vi "Teleop.vi"(10 "Match Info":T1={"Autonomous Elapsed Seconds"=0.0, "TeleOp Elapsed Seconds"=0.0, "Disabled Elapsed Seconds"=0.0, "Visited Autonomous"=FALSE, "Visited TeleOp"=FALSE, "Visited Disabled"=FALSE, "Autonomous Settings"={"Autonomous Style"=enum."Independent", "VI Refnum"=refnum}}, 11 "Call Context":T2) -> ()   [LabVIEW 2016]
doc: "This VI is called for each TeleOp packet received from the DS where the robot is not disabled. It is often used to read from the joysticks and update I/O or to update setpoints for timed control loops. It should complete and return within 20 milliseconds or it may miss DS packets."
uses:
  <vilib>/Rock Robotics/WPI/DriverStation/WPI_DriverStationDerivedRobotMode.ctl
  <vilib>/Rock Robotics/WPI/DriverStation/WPI_DriverStationMatch Info.ctl
  <vilib>/Rock Robotics/WPI/Utilities/WPI_GetSetVariantRefNum.vi
  <vilib>/Rock Robotics/Network Tables/NT Write Boolean Array.vi
  <vilib>/Rock Robotics/Network Tables/NT Write Numeric Array.vi
  <vilib>/Rock Robotics/Network Tables/NT Read Boolean.vi
  <vilib>/Rock Robotics/Network Tables/NT Read Number.vi
  Robot Global Data.vi
  <vilib>/Rock Robotics/Network Tables/NT Write Boolean.vi
panel:
  out "servoRotation":dbl
  out "element 2":dbl
  out "Boolean 2":bool
  out "Boolean":bool
  out "Sample Slider 0":dbl(slide) scale=0.0..5.0
  out "Sample Boolean 1":bool
  out "Sample Boolean 0":bool
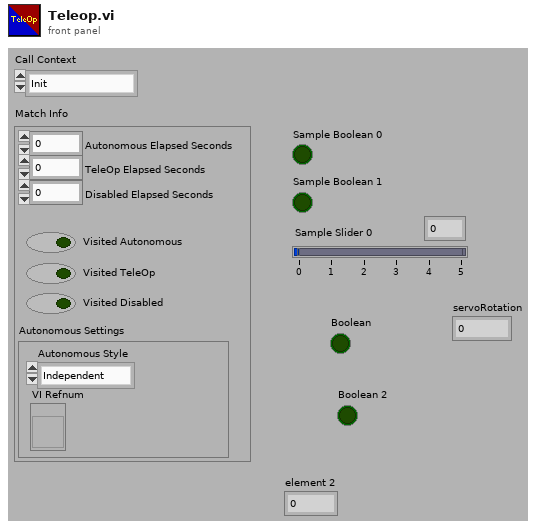
[diagram p1: front panel]
types:
  T1 = typedef "WPI_DriverStationMatch Info.ctl" = cluster{"Autonomous Elapsed Seconds":dbl, "TeleOp Elapsed Seconds":dbl, "Disabled Elapsed Seconds":dbl, "Visited Autonomous":bool, "Visited TeleOp":bool, "Visited Disabled":bool, "Autonomous Settings":cluster{"Autonomous Style":enum16{"Iterative", "Independent"}, "VI Refnum":refnum<vi>}}
  T2 = typedef "WPI_DriverStationDerivedRobotMode.ctl" = enum16{"Init", "Execute", "Stop"}
  T3 = typedef "WPI_RobotDriveDevRef.ctl" = cluster{"DevStatus":errorcluster, "Motors[]":T4[], "Square Inputs":bool, "Max Output":dbl}
  T4 = typedef "WPI_MotorControlDeviceRef.ctl" = cluster{"DeviceStatus":errorcluster, "Type":T5, "PWM":cluster{"PWM Channel":T6, "DeadBand":T7}, "CAN":cluster{"Device Number":u8, "SetOutput VI Ref":variant, "GetOutput VI Ref":variant, "Enable VI Ref":variant, "Disable VI Ref":variant, "Data":variant}, "Invert":bool}
  T5 = typedef "WPI_MotorControlType.ctl" = enum16{"PWM", "CAN"}
  T6 = typedef "FPGA_DIOPWMChannel.ctl" = enum8{"PWM 0", "PWM 1", "PWM 2", "PWM 3", "PWM 4", "PWM 5", "PWM 6", "PWM 7", "PWM 8", "PWM 9", "PWM MXP 0", "PWM MXP 1", "PWM MXP 2", "PWM MXP 3", "PWM MXP 4", "PWM MXP 5", "PWM MXP 6", "PWM MXP 7", "PWM MXP 8", "PWM MXP 9", "Invalid"}
  T7 = typedef "WPI_PWMDeadband.ctl" = cluster{"Name":string, "maxPositivePwm":i32, "minPositivePwm":i32, "centerPwm":i32, "maxNegativePwm":i32, "minNegativePwm":i32, "angularRange":u16}
  T8 = typedef "WPI_JoystickDevRef.ctl" = cluster{"Device":T9}
  T9 = typedef "WPI_JoystickDeviceEnum.ctl" = enum16{"USB 0", "USB 1", "USB 2", "USB 3", "USB 4", "USB 5"}
  T10 = cluster{"Buttons[0]":bool, "Buttons[1]":bool, "Buttons[2]":bool, "Buttons[3]":bool, "Buttons[4]":bool, "Buttons[5]":bool, "Buttons[6]":bool, "Buttons[7]":bool, "Buttons[8]":bool}
  T11 = typedef "WPI_ServoDeviceRef.ctl" = cluster{"DeviceStatus":errorcluster, "PWM Channel":T6, "DeadBand":T7}
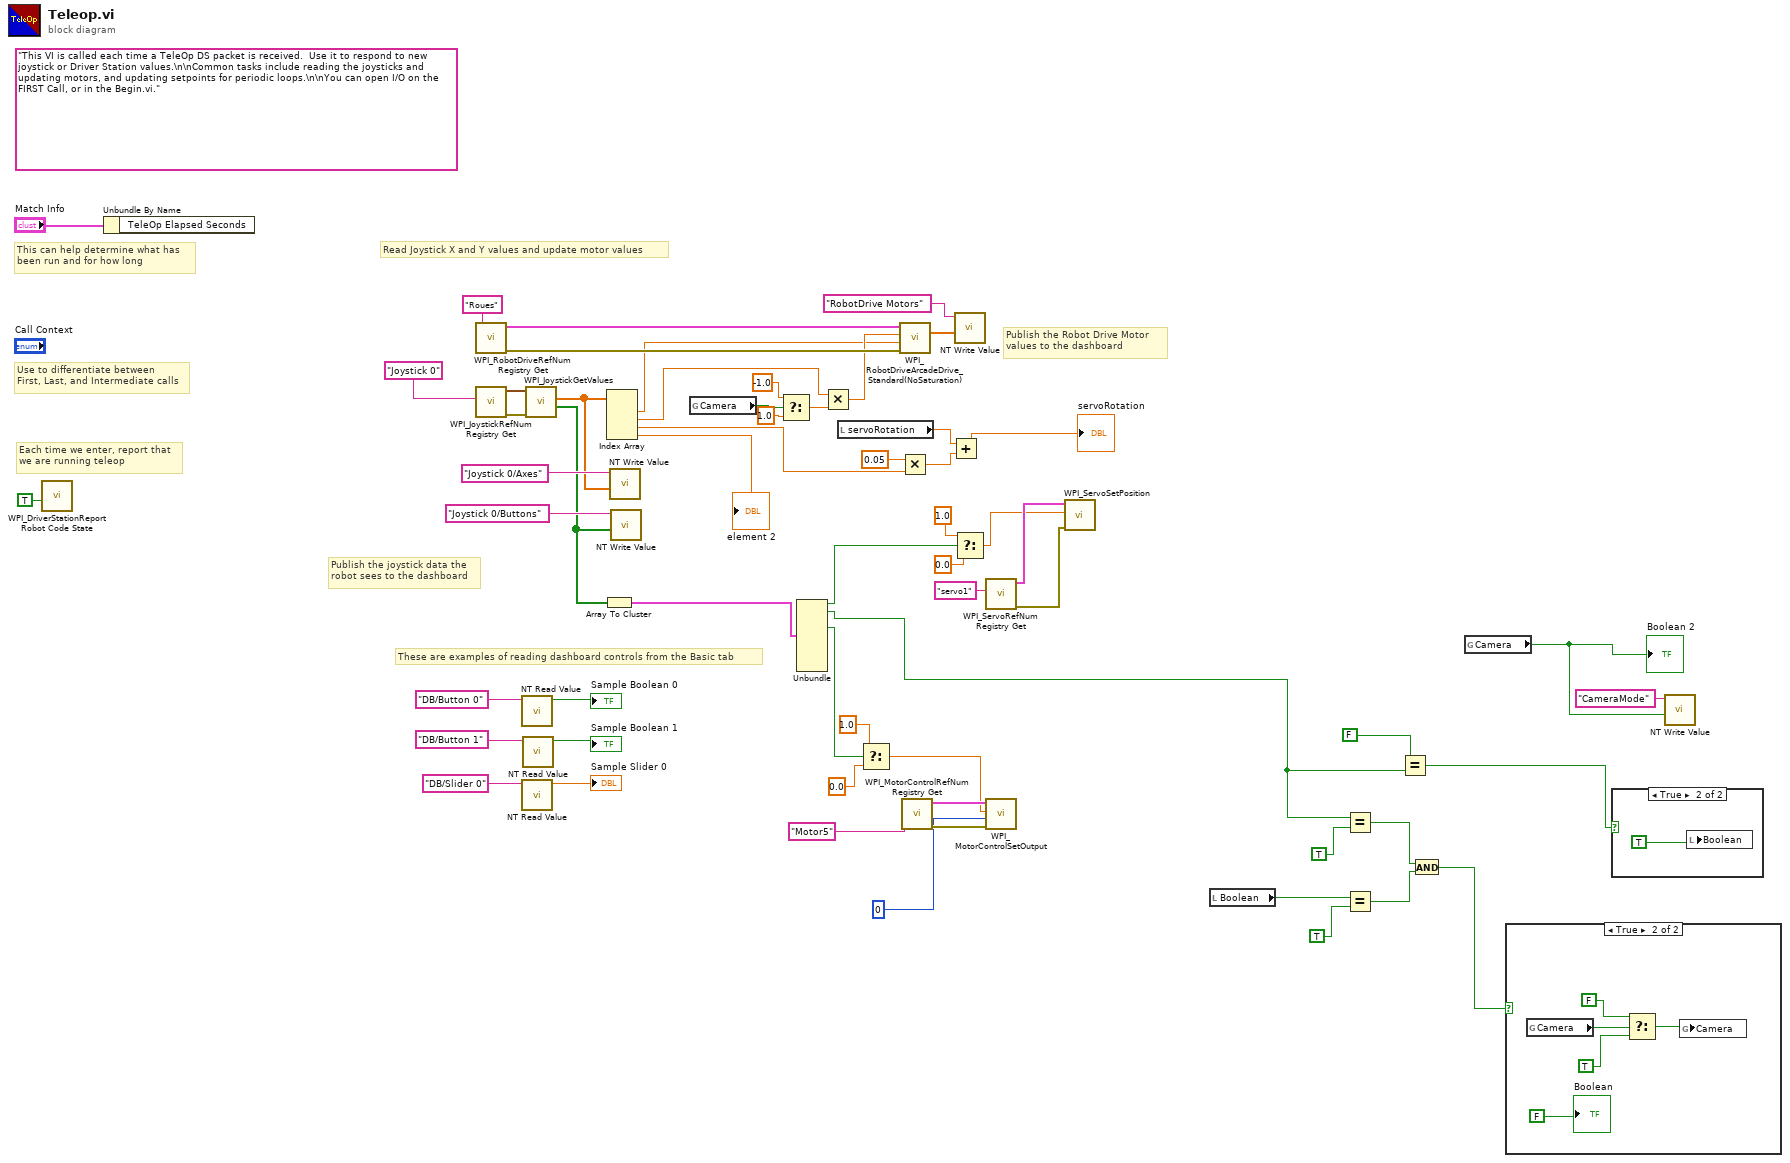
[diagram p0: block diagram]
diagram:
  (unwired) "This VI is called each time a TeleOp DS packet is received.  Use it to respond to new joystick or Driver Station values.\n\nCommon tasks include reading the joysticks and updating motors, and updating setpoints for periodic loops.\n\nYou can open I/O on the FIRST Call, or in the Begin.vi."
  # "These are examples of reading dashboard controls from the Basic tab"
  # "Publish the Robot Drive Motor\nvalues to the dashboard"
  # "Publish the joystick data the\nrobot sees to the dashboard"
  # "Each time we enter, report that\nwe are running teleop"
  # "Use to differentiate between\nFirst, Last, and Intermediate calls"
  # "This can help determine what has\nbeen run and for how long"
  # "Read Joystick X and Y values and update motor values"
  n1 = call <vilib>:"WPI_DriverStationReport Robot Code State.vi"("TeleOp"=TRUE ("Autonomous")) -> ()  [unwired: 10 in, 1 out]
  n2 = Unbundle By Name("Match Info") -> ()  [unwired: 1 out]
  n3 = call <vilib>:"WPI_RobotDriveRefNum Registry Get.vi"("refnum name"="Roues") -> ("error out"=w43:errorcluster, "RobotDriveDevRef"=w58:T3)  [unwired: 1 in, 8 out]
  n4 = call <vilib>:"WPI_JoystickRefNum Registry Get.vi"("refnum name"="Joystick 0") -> ("error out"=w16:errorcluster, "JoystickDevRef"=w56:T8)  [unwired: 1 in, 8 out]
  n5 = call-poly <vilib>:"NT Read Value.vi"("Name"="DB/Button 0" ("refnum name")) -> ("Boolean"=→"Sample Boolean 0":bool)  [unwired: 9 in, 1 out]
  n6 = call-poly <vilib>:"NT Read Value.vi"("Name"="DB/Slider 0" ("refnum name")) -> ("Numeric"=→"Sample Slider 0":dbl)  [unwired: 9 in, 1 out]
  n7 = call-poly <vilib>:"NT Read Value.vi"("Name"="DB/Button 1" ("refnum name")) -> ("Boolean"=→"Sample Boolean 1":bool)  [unwired: 9 in, 1 out]
  n8 = call <vilib>:"WPI_JoystickGetValues.vi"("error in (no error)"=w16, "JoystickDevRef"=w56) -> ("Buttons"=w42:bool[], "Axes"=w52:dbl[])  [unwired: 5 in, 3 out]
  n9 = Array To Cluster(array=w42) -> (cluster=w41:T10)
  n10 = Index Array(array=w52) -> (element #1=w11:dbl, element #2=w13:dbl, element #3=w9:dbl, element #4=→"element 2":dbl)  [unwired: 4 in]
  n11 = call-poly <vilib>:"NT Write Value.vi"("Numeric Array"=w52, "Name"="Joystick 0/Axes") -> ()  [unwired: 9 in, 1 out]
  n12 = call-poly <vilib>:"NT Write Value.vi"("Boolean Array"=w42, "Name"="Joystick 0/Buttons") -> ()  [unwired: 9 in, 1 out]
  n13 = global read "Robot Global Data.vi" "Camera"() -> (w18:bool)
  n14 = Select(t=-1.0, s=w18, f=1.0) -> (s? t:f=w14:dbl)
  n15 = Unbundle(w41) -> ("Buttons[0]"=w1:bool, "Buttons[1]"=w29:bool, "Buttons[3]"=w28:bool)  [unwired: 6 out]
  n16 = Multiply(x=w13, y=w14) -> (x*y=w12:dbl)
  n17 = local read "servoRotation"() -> (w7:dbl)
  n18 = Select(t=1.0, s=w28, f=0.0) -> (s? t:f=w23:dbl)
  n19 = call <vilib>:"WPI_RobotDriveArcadeDrive_Standard(NoSaturation).vi"("error in (no error)"=w43, "Y axis value"=w11, "X axis value"=w12, "RobotDriveDevRef"=w58) -> ("Motor Values"=w45:dbl[])  [unwired: 7 out]
  n20 = Multiply(x=0.05, y=w9) -> (x*y=w6:dbl)
  n21 = call <vilib>:"WPI_MotorControlRefNum Registry Get.vi"("refnum name"="Motor5") -> ("error out"=w25:errorcluster, "MotorControlDevRef"=w26:T4)  [unwired: 9 in]
  n22 = Add(x=w7, y=w6) -> (x+y=→"servoRotation":dbl)
  n23 = call-poly <vilib>:"NT Write Value.vi"("Numeric Array"=w45, "Name"="RobotDrive Motors") -> ()  [unwired: 9 in, 1 out]
  n24 = Select(t=1.0 ("upper limit"), s=w1, f=0.0 ("lower limit")) -> (s? t:f=w2:dbl)
  n25 = call <vilib>:"WPI_ServoRefNum Registry Get.vi"("refnum name"="servo1") -> ("error out"=w38:errorcluster, "ServoDeviceRef"=w40:T11)  [unwired: 9 in]
  n26 = call <vilib>:"WPI_MotorControlSetOutput.vi"("error in (no error)"=w25, "options"=u8 0, "Output"=w23, "MotorControlDevRef"=w26) -> ()  [unwired: 5 in, 3 out]
  n27 = call <vilib>:"WPI_ServoSetPosition.vi"("error in (no error)"=w38, "Position"=w2, "ServoDeviceRef"=w40) -> ()  [unwired: 7 in, 2 out]
  n28 = local read "Boolean"() -> (w36:bool)
  n29 = Equal?(x=w29, y=TRUE) -> (x = y?=w34:bool)
  n30 = Equal?(x=w36, y=TRUE) -> (x = y?=w33:bool)
  n31 = Equal?(x=FALSE, y=w29) -> (x = y?=w30:bool)
  n32 = And(x=w34, y=w33) -> (x .and. y?=w32:bool)
  n33 = global read "Robot Global Data.vi" "Camera"() -> (w20:bool)
  "Boolean 2" <- w20
  n34 = case shown="True" w32 {
    frame False {
    }
    frame True {
      n35 = global read "Robot Global Data.vi" "Camera"() -> (w64:bool)
      n36 = Select(t=FALSE, s=w64, f=TRUE) -> (s? t:f=w63:bool)
      n37 = global write "Robot Global Data.vi" "Camera"(w63) -> ()
      "Boolean" <- FALSE
    }
  }
  n38 = case shown="True" w30 {
    frame False {
    }
    frame True {
      n39 = local write "Boolean"(TRUE) -> ()
    }
  }
  n40 = call-poly <vilib>:"NT Write Value.vi"("Boolean"=w20, "Name"="CameraMode") -> ()  [unwired: 9 in, 1 out]
